vi "Create Configuration Source Distribution.vi"(4 "Base Path":path, 6 "Extra Page Names":string[](array[string]), 7 "XML File Refnum":refnum<vi>, 8 "error in (no error)":errorcluster, 9 "Library Refnum":refnum<vi>, 10 "Project Refnum":refnum<vi>, 11 "Custom Device Name":string) -> (0 "error out":errorcluster)   [LabVIEW 2020, in "Custom Device Template Tool.lvlib"]
uses:
  <vilib>/NI VeriStand/Custom Device Tools/Custom Device Template Tool/Custom Device Template Tool.lvlib
  <vilib>/AppBuilder/AB_API/common/AB_API Default Destinations.ctl
  <vilib>/AppBuilder/AB_API/common/AB_API Path Exclusions.ctl
  <vilib>/AppBuilder/AB_API/common/AB_API Primary Exclusions.ctl
  <vilib>/AppBuilder/AB_API/common/AB_API Destination Type.ctl
  <vilib>/AppBuilder/AB_API/SDIST/NI_AB_API_SDIST.lvclass
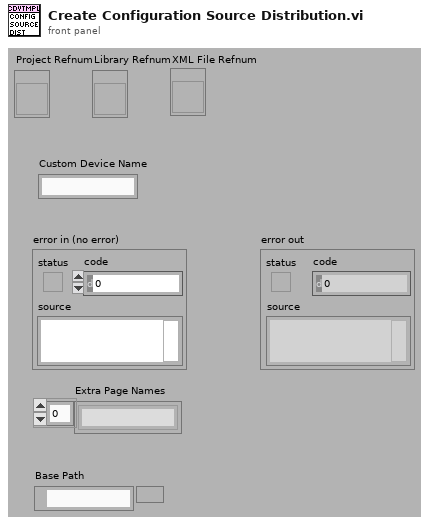
[diagram p1: front panel]
types:
  T1 = typedef "AB_API Default Destinations.ctl" = enum16{"Destination Directory", "Support Directory"}
  T2 = typedef "AB_API Path Exclusions.ctl" = cluster{"Exclude files from vi.lib":bool, "Exclude files from instr.lib":bool, "Exclude files from user.lib":bool}
  T3 = typedef "AB_API Primary Exclusions.ctl" = cluster{"Disconnect type definitions":bool, "Remove unused polymorphic VI instances":bool, "Remove unused members of project libraries":bool, "Modify project library file after removing unused members":bool}
  T4 = typedef "AB_API Destination Type.ctl" = enum16{"directory", "directory (preserve hierarchy)", "LLB"}
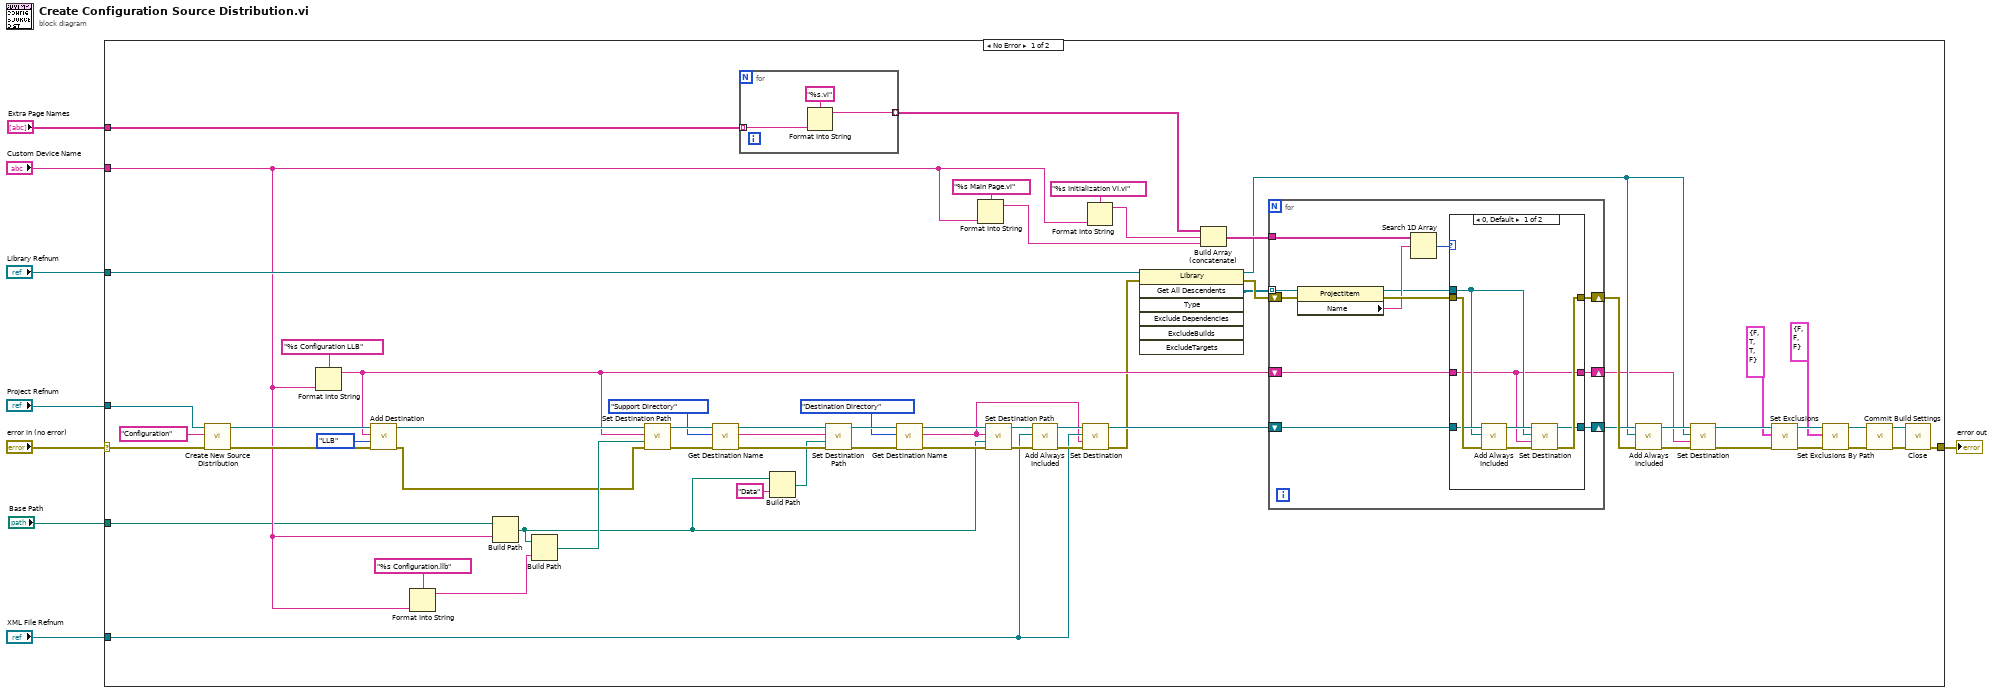
[diagram p0: block diagram]
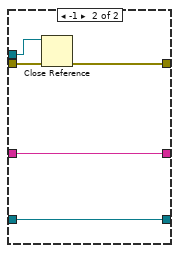
[diagram p2: hidden frame]
diagram:
  n1 = case shown="No Error" "error in (no error)" {
    selector: "error in (no error)" -> [w65 w101]
    tunnel: [w32 w101] -> w8
    tunnel: "Project Refnum" -> [w64 _]
    tunnel: "Library Refnum" -> [w62 _]
    tunnel: "Custom Device Name" -> [w48 _]
    tunnel: "XML File Refnum" -> [w37 _]
    tunnel: "Extra Page Names" -> [w23 _]
    tunnel: "Base Path" -> [w20 _]
    frame No Error {
      n2 = call <vilib>:"Create New Source Distribution.vi"("error in (no error)"=w65, "Build specification name"="Configuration", "Project Refnum"=w64) -> ("error out"=w52:errorcluster, "SDIST out"=w68:refnum<class "NI_AB_API_SDIST.lvclass">)  [unwired: 7 in]
      n3 = Format Into String(format string="%s Configuration LLB", w48) -> (resulting string=w46:string)  [unwired: 2 in, 1 out]
      n4 = call-dynamic "Add Destination.vi"("error in (no error)"=w52, "Destination type (directory)"=AB_API_Destination_Type."LLB", "Destination label"=w46, "SDIST in"=w68) -> ("error out"=w21:errorcluster, "SDIST out"=w54:refnum<class "NI_AB_API_SDIST.lvclass">)  [unwired: 6 in]
      n5 = Format Into String(format string="%s Configuration.llb", w48) -> (resulting string=w49:string)  [unwired: 2 in, 1 out]
      n6 = Build Path(base path=w20, name or relative path=w48) -> (appended path=w19:path)
      n7 = Build Path(base path=w19, name or relative path=w49) -> (appended path=w47:path)
      n8 = call-dynamic "Set Destination Path.vi"("error in (no error)"=w21, "Destination path"=w47, "Destination label"=w46, "SDIST in"=w54) -> ("error out"=w14:errorcluster, "SDIST out"=w16:refnum<class "NI_AB_API_SDIST.lvclass">)  [unwired: 6 in]
      n9 = call-dynamic "Get Destination Name.vi"("error in (no error)"=w14, "Default Destinations"=AB_API_Default_Destinations."Support Directory", "SDIST in"=w16) -> ("error out"=w69:errorcluster, "Destination Name"=w12:string, "SDIST out"=w13:refnum<class "NI_AB_API_SDIST.lvclass">)  [unwired: 6 in]
      n10 = for {
        tunnel: w23 -> [w74] mode=indexing
        tunnel: [w73] -> w22 mode=indexing
        n11 = Format Into String(format string="%s.vi", w74) -> (resulting string=w73:string)  [unwired: 2 in, 1 out]
      }
      n12 = Build Path(base path=w19, name or relative path="Data") -> (appended path=w17:path)
      n13 = call-dynamic "Set Destination Path.vi"("error in (no error)"=w69, "Destination path"=w17, "Destination label"=w12, "SDIST in"=w13) -> ("error out"=w10:errorcluster, "SDIST out"=w70:refnum<class "NI_AB_API_SDIST.lvclass">)  [unwired: 6 in]
      n14 = call-dynamic "Get Destination Name.vi"("error in (no error)"=w10, "Default Destinations"=AB_API_Default_Destinations."Destination Directory", "SDIST in"=w70) -> ("error out"=w72:errorcluster, "Destination Name"=w9:string, "SDIST out"=w71:refnum<class "NI_AB_API_SDIST.lvclass">)  [unwired: 6 in]
      n15 = Format Into String(format string="%s Main Page.vi", w48) -> (resulting string=w57:string)  [unwired: 2 in, 1 out]
      n16 = call-dynamic "Set Destination Path.vi"("error in (no error)"=w72, "Destination path"=w19, "Destination label"=w9, "SDIST in"=w71) -> ("error out"=w38:errorcluster, "SDIST out"=w39:refnum<class "NI_AB_API_SDIST.lvclass">)  [unwired: 6 in]
      n17 = call-dynamic "Add Always Included.vi"("error in (no error)"=w38, "ProjectItem Refnum"=w37, "SDIST in"=w39) -> ("error out"=w41:errorcluster, "SDIST out"=w40:refnum<class "NI_AB_API_SDIST.lvclass">)  [unwired: 7 in]
      n18 = call-dynamic "Set Destination.vi"("error in (no error)"=w41, "Destination label"=w9, "ProjectItem Refnum"=w37, "SDIST in"=w40) -> ("error out"=w35:errorcluster, "SDIST out"=w36:refnum<class "NI_AB_API_SDIST.lvclass">)  [unwired: 6 in]
      n19 = Format Into String(format string="%s Initialization VI.vi", w48) -> (resulting string=w58:string)  [unwired: 2 in, 1 out]
      n20 = invoke class="Library" method="Get All Descendents"(reference=w62, error in=w35) -> (reference out=w43:refnum<vi>, error out=w66:errorcluster, "All Descendents"=w61:refnum<vi>[])  [unwired: 5 in, 4 out]
      n21 = Build Array (concatenate)(w22, w58, w57) -> (w56:string[])
      n22 = for {
        tunnel: w61 -> [w86] mode=indexing
        shift-right: [w80] -> w67
        shift-left: w66 -> [w85]
        tunnel: w56 -> [w84]
        shift-right: [w78] -> w55
        shift-left: w36 -> [w79]
        shift-right: [w76] -> w42
        shift-left: w46 -> [w77]
        n23 = property class="ProjectItem"(reference=w86, error in=w85) -> (reference out=w81:refnum<vi>, error out=w87:errorcluster, "Name"=w83:string)
        n24 = Search 1D Array(1D array=w84, element=w83) -> (index of element=w82:i32)  [unwired: 1 out]
        n25 = case shown="0, Default" w82 {
          tunnel: w87 -> [w95 w100]
          tunnel: w81 -> [w89 w99]
          tunnel: [w91 w98] -> w80
          tunnel: w79 -> [w94 w97]
          tunnel: [w90 w97] -> w78
          tunnel: w77 -> [w88 w96]
          tunnel: [w88 w96] -> w76
          frame 0, Default {
            n26 = call-dynamic "Add Always Included.vi"("error in (no error)"=w95, "ProjectItem Refnum"=w89, "SDIST in"=w94) -> ("error out"=w92:errorcluster, "SDIST out"=w93:refnum<class "NI_AB_API_SDIST.lvclass">)  [unwired: 7 in]
            n27 = call-dynamic "Set Destination.vi"("error in (no error)"=w92, "Destination label"=w88, "ProjectItem Refnum"=w89, "SDIST in"=w93) -> ("error out"=w91:errorcluster, "SDIST out"=w90:refnum<class "NI_AB_API_SDIST.lvclass">)  [unwired: 6 in]
          }
          frame -1 {
            n28 = Close Reference(reference=w99, error in (no error)=w100) -> (error out=w98:errorcluster)
          }
        }
      }
      n29 = call-dynamic "Add Always Included.vi"("error in (no error)"=w67, "ProjectItem Refnum"=w43, "SDIST in"=w55) -> ("error out"=w45:errorcluster, "SDIST out"=w44:refnum<class "NI_AB_API_SDIST.lvclass">)  [unwired: 7 in]
      n30 = call-dynamic "Set Destination.vi"("error in (no error)"=w45, "Destination label"=w42, "ProjectItem Refnum"=w43, "SDIST in"=w44) -> ("error out"=w30:errorcluster, "SDIST out"=w31:refnum<class "NI_AB_API_SDIST.lvclass">)  [unwired: 6 in]
      n31 = call-dynamic "Set Exclusions.vi"("error in (no error)"=w30, "Exclusions"=T3 {"Disconnect type definitions"=FALSE, "Remove unused polymorphic VI instances"=TRUE, "Remove unused members of project libraries"=TRUE, "Modify project library file after removing unused members"=FALSE}, "SDIST in"=w31) -> ("error out"=w27:errorcluster, "SDIST out"=w28:refnum<class "NI_AB_API_SDIST.lvclass">)  [unwired: 7 in]
      n32 = call-dynamic "Set Exclusions By Path.vi"("error in (no error)"=w27, "Path exclusions"=T2 {"Exclude files from vi.lib"=FALSE, "Exclude files from instr.lib"=FALSE, "Exclude files from user.lib"=FALSE}, "SDIST in"=w28) -> ("error out"=w25:errorcluster, "SDIST out"=w26:refnum<class "NI_AB_API_SDIST.lvclass">)  [unwired: 7 in]
      n33 = call-dynamic "Commit Build Settings.vi"("error in (no error)"=w25, "SDIST in"=w26) -> ("error out"=w33:errorcluster, "SDIST out"=w34:refnum<class "NI_AB_API_SDIST.lvclass">)  [unwired: 8 in]
      n34 = call-dynamic "Close.vi"("error in (no error)"=w33, "SDIST in"=w34) -> ("error out"=w32:errorcluster)  [unwired: 9 in]
    }
    frame Error {
    }
  }
  "error out" <- w8
